vi "rad_Get AppImage From Target.vi"(7 "Temp Folder":path, 8 "error in (no error)":errorcluster, 11 "Target settings":T4={"Hostname"="", "Serial number"="", "Product name"="", "Product code"=0, "System status"="", "Credential type"=enum."None/Unlocked", "User added?"=FALSE, "Primary NIC"={"MAC address"="", "IP Address Request Mode"=2, "IP address"="", "Subnet mask"="", "Gateway"="", "DNS server"=""}} {"Primary NIC"."IP Address Request Mode" items=["Static"=1, "DHCP/Link-Local"=2, "Link-Local Only"=4, "DHCP Only"=8]}) -> (0 "error out":errorcluster, 2 "Supports System\nConfig Metadata":bool, 3 "AppImage Properties":T1)   [LabVIEW 2014]
uses:
  Targets/TypeDefs/rad_Target Information.ctl
  Targets/TypeDefs/rad_Target Network Settings.ctl
  TypeDefs/rad_Application Image Properties.ctl
  TypeDefs/rad_FPGA Properties.ctl
  TypeDefs/rad_FPGA Flash Properties.ctl
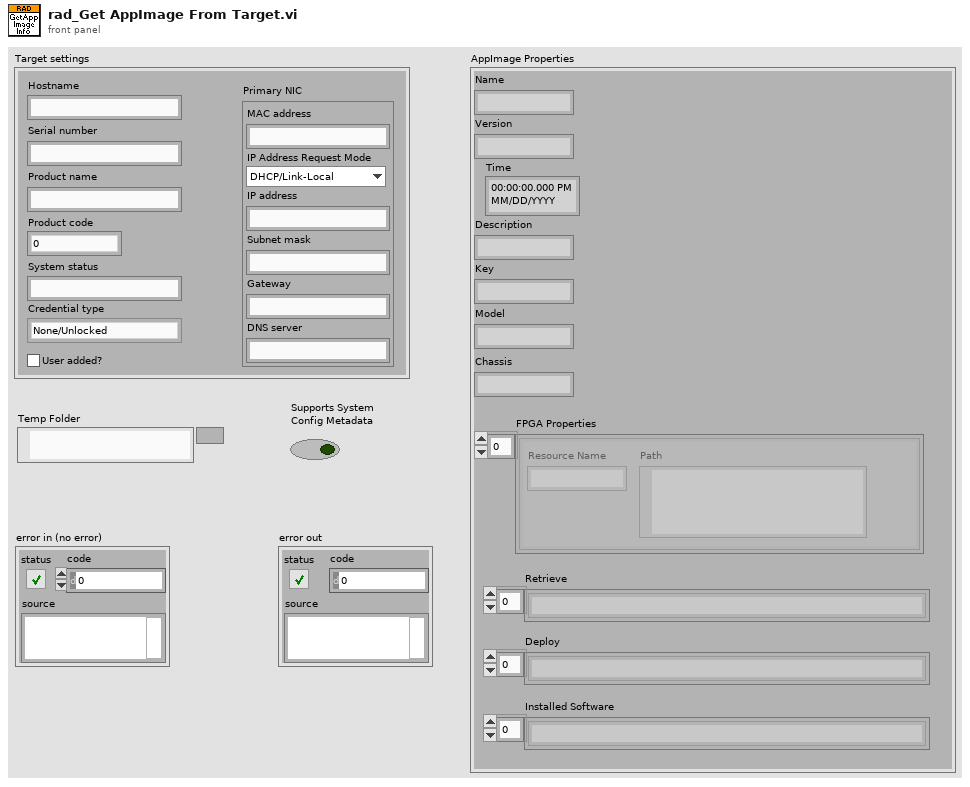
[diagram p1: front panel]
types:
  T1 = typedef "rad_Application Image Properties.ctl" = cluster{"Name":string, "Version":string, "Time":timestamp, "Description":string, "Key":string, "Chassis":string, "FPGA Properties":T2, "Model":string, "Retrieve":string[], "Deploy":string[], "Installed Software":string[]}
  T2 = typedef "rad_FPGA Properties.ctl" = T3[]
  T3 = typedef "rad_FPGA Flash Properties.ctl" = cluster{"Resource Name":string, "Path":path}
  T4 = typedef "rad_Target Information.ctl" = cluster{"Hostname":string, "Serial number":string, "Product name":string, "Product code":i32, "System status":string, "Credential type":enum16{"None/Unlocked", "FTP Password", "NIAuth Credentials"}, "User added?":bool, "Primary NIC":T5}
  T5 = typedef "rad_Target Network Settings.ctl" = cluster{"MAC address":string, "IP Address Request Mode":i32, "IP address":string, "Subnet mask":string, "Gateway":string, "DNS server":string}
  T6 = typedef "nisyscfg.lvlib/Software 1.2.ctl" = cluster{"title":string, "description":string, "ID":string, "version":string, "component type":T7}
  T7 = typedef "nisyscfg.lvlib/Component Type.ctl" = u32
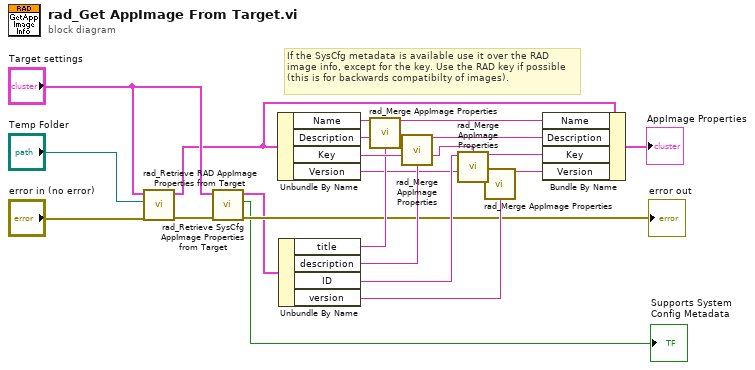
[diagram p0: block diagram]
diagram:
  # "If the SysCfg metadata is available use it over the RAD image info, except for the key. Use the RAD key if possible (this is for backwards compatibilty of images)."
  n1 = call "rad_Retrieve RAD AppImage Properties from Target.vi"("error in (no error)"="error in (no error)", "App Images Temp Folder"="Temp Folder", "Target settings"="Target settings") -> ("error out"=w3:errorcluster, "RAD AppImage Properties"=w10:T1)  [unwired: 7 in]
  n2 = call "rad_Retrieve SysCfg AppImage Properties from Target.vi"("error in (no error)"=w3, "Target settings"="Target settings") -> ("error out"=→"error out":errorcluster, "Supports System\nConfig Metadata"=→"Supports System\nConfig Metadata":bool, "image metadata"=w4:T6)  [unwired: 7 in]
  n3 = Unbundle By Name(w10) -> ("Name"=w5:string, "Description"=w8:string, "Key"=w19:string, "Version"=w9:string)
  n4 = Unbundle By Name(w4) -> ("title"=w12:string, "description"=w13:string, "ID"=w18:string, "version"=w14:string)
  n5 = call "rad_Merge AppImage Properties.vi"("RAD property"=w5, "SysCfg property"=w12) -> ("New Property"=w15:string)  [unwired: 13 in]
  n6 = call "rad_Merge AppImage Properties.vi"("RAD property"=w8, "SysCfg property"=w13) -> ("New Property"=w16:string)  [unwired: 13 in]
  n7 = call "rad_Merge AppImage Properties.vi"("RAD property"=w18, "SysCfg property"=w19) -> ("New Property"=w17:string)  [unwired: 13 in]
  n8 = call "rad_Merge AppImage Properties.vi"("RAD property"=w9, "SysCfg property"=w14) -> ("New Property"=w11:string)  [unwired: 13 in]
  n9 = Bundle By Name(cluster=w10, "Name"=w15, "Description"=w16, "Key"=w17, "Version"=w11) -> (→"AppImage Properties":T1)
